vi "PMTRunPulseSet.vi"(3 "error in":errorcluster, 4 "Cluster":T1) -> (0 "error out":errorcluster, 1 "times":u32[][](array[numeric]), 2 "counts":cluster{u32[], u32[], u32[], u32[]})   [LabVIEW 2017]
uses:
  <vilib>/rvi/interface/nirviMethod/nirviMethod.xnode
  <vilib>/rvi/interface/nirviReadWriteControl/nirviReadWriteControl.xnode
  NiFpgaLv.dll
  <vilib>/Utility/error.llb/Error Cluster From Error Code.vi
  <vilib>/rvi/interface/Simulation/niFpgaSimulationCallBeginRW.vi
  <vilib>/rvi/errors/niLvFpgaAdjustHostInterfaceError.vi
  <vilib>/FPGAPlugInAG/Dynamic/niLvFpga_ReadFifo_Dynamic.vi
  <vilib>/rvi/errors/niLvFpgaMergeErrorWithErrorCode.vi
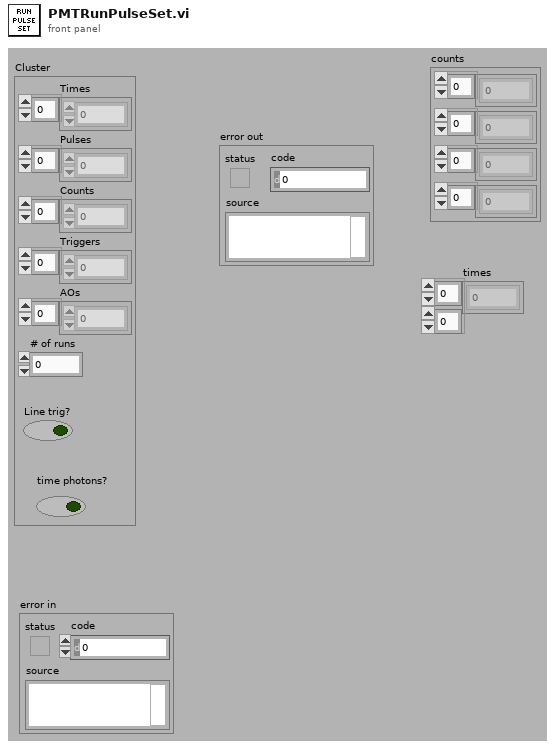
[diagram p1: front panel]
types:
  T1 = cluster{"Times":u32[], "Pulses":u64[], "Counts":u8[], "Triggers":u8[], "AOs":u8[], "# of runs":i32, "Line trig?":bool, "time photons?":bool}
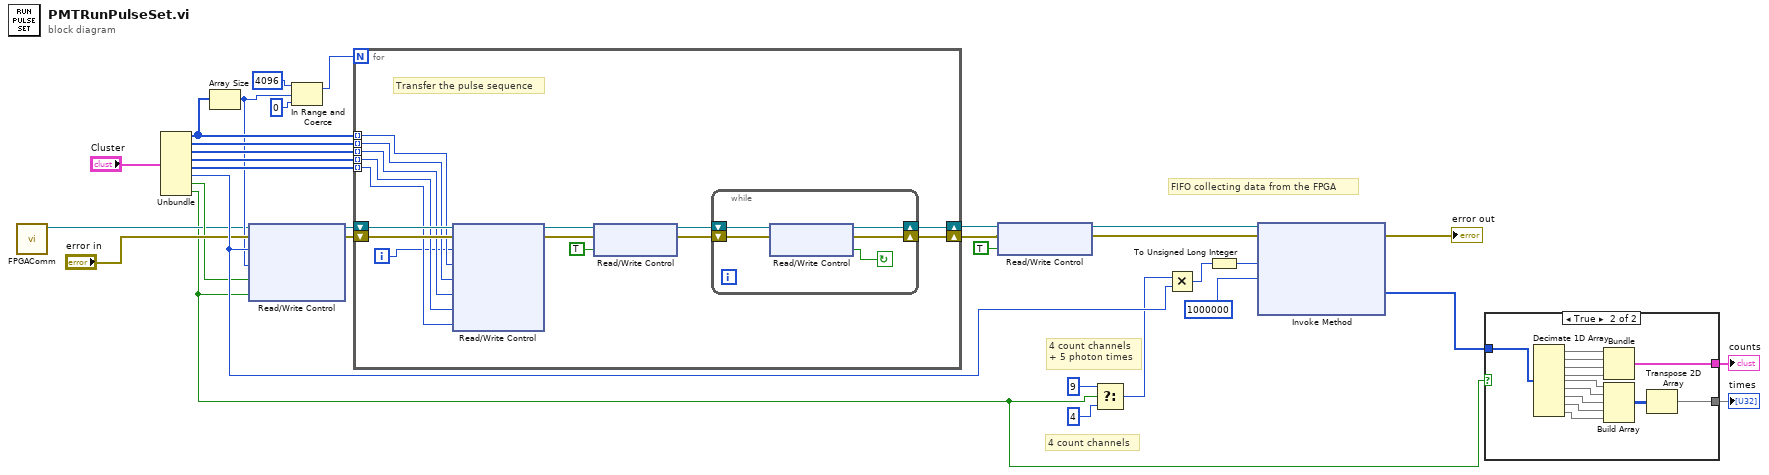
[diagram p0: block diagram]
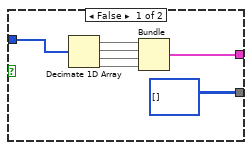
[diagram p2: hidden frame]
diagram:
  # "4 count channels\n+ 5 photon times"
  # "4 count channels"
  # "FIFO collecting data from the FPGA"
  n1 = call "FPGAComm.vi"() -> ("FPGA VI Reference Out 2"=w8:refnum<k20>)  [unwired: 6 in, 1 out]
  n2 = Unbundle("Cluster") -> ("Times"=w11:u32[], "Pulses"=w25:u64[], "Counts"=w26:u8[], "Triggers"=w27:u8[], "AOs"=w28:u8[], "# of runs"=w32:i32, "Line trig?"=w9:bool, "time photons?"=w4:bool)
  n3 = Array Size(array=w11) -> (size(s)=w10:i32)
  n4 = xnode "Read/Write Control"("FPGA VI Reference In"=w8, "error in"="error in", "# of runs"=w32, "# of pulses"=w10, "Line trig?"=w9, "Send photons?"=w4) -> ("FPGA VI Reference Out"=w29:refnum<k20>, "error out"=w31:errorcluster)
  n5 = In Range and Coerce(upper limit=4096, x=w10, lower limit=0) -> (coerced(x)=w24:i32)  [unwired: 1 out]
  n6 = for {
    N: w24 -> [_]
    tunnel: w11 -> [w45] mode=indexing
    tunnel: w25 -> [w44] mode=indexing
    tunnel: w26 -> [w43] mode=indexing
    tunnel: w27 -> [w42] mode=indexing
    tunnel: w28 -> [w41] mode=indexing
    shift-right: [w35] -> w18
    shift-left: w29 -> [w47]
    shift-right: [w34] -> w19
    shift-left: w31 -> [w46]
    i -> [w33]
    # "Transfer the pulse sequence"
    n7 = xnode "Read/Write Control"("FPGA VI Reference In"=w47, "error in"=w46, "pulse number"=w33, "time data"=w45, "digout data"=w44, "count data"=w43, "trigger data"=w42, "AO data"=w41) -> ("FPGA VI Reference Out"=w39:refnum<k20>, "error out"=w38:errorcluster)
    n8 = xnode "Read/Write Control"("FPGA VI Reference In"=w39, "error in"=w38, "data waiting"=TRUE) -> ("FPGA VI Reference Out"=w37:refnum<k20>, "error out"=w36:errorcluster)
    n9 = while {
      shift-right: [w50] -> w35
      shift-left: w37 -> [w52]
      shift-right: [w49] -> w34
      shift-left: w36 -> [w51]
      stop <- w48 continue-if-true
      n10 = xnode "Read/Write Control"("FPGA VI Reference In"=w52, "error in"=w51) -> ("FPGA VI Reference Out"=w50:refnum<k20>, "error out"=w49:errorcluster, "data waiting"=w48:bool)
    }
  }
  n11 = xnode "Read/Write Control"("FPGA VI Reference In"=w18, "error in"=w19, "start sequence"=TRUE) -> ("FPGA VI Reference Out"=w12:refnum<k20>, "error out"=w13:errorcluster)
  n12 = Select(t=9, s=w4, f=4 ("x")) -> (s? t:f=w6:i32)
  n13 = Multiply(x=w6, y=w32) -> (x*y=w15:i32)
  n14 = To Unsigned Long Integer(number=w15) -> (unsigned 32bit integer=w17:u32)
  n15 = xnode "Invoke Method"("FPGA VI Reference In"=w12, "error in"=w13, "Number of Elements"=w17, "Timeout (ms)"=1000000) -> ("error out"=→"error out":errorcluster, "Data"=w3:u32[])  [unwired: 2 out]
  n16 = case shown="True" w4 {
    tunnel: w3 -> [w59 w68]
    tunnel: [w54 w67] -> w2
    tunnel: [u32[][] [] ("transposed array") w60] -> w1
    frame False {
      n17 = Decimate 1D Array(w59) -> (w58:u32[], w57:u32[], w56:u32[], w55:u32[])
      n18 = Bundle(w58, w57, w56, w55) -> (w54:cluster{u32[], u32[], u32[], u32[]})  [unwired: 1 in]
    }
    frame True {
      n19 = Decimate 1D Array(w68) -> (w72:u32[], w71:u32[], w70:u32[], w69:u32[], w66:u32[], w65:u32[], w64:u32[], w63:u32[], w62:u32[])
      n20 = Bundle(w72, w71, w70, w69) -> (w67:cluster{u32[], u32[], u32[], u32[]})  [unwired: 1 in]
      n21 = Build Array(w66, w65, w64, w63, w62) -> (w61:u32[][])
      n22 = Transpose 2D Array(2D array=w61) -> (transposed array=w60:u32[][])
    }
  }
  "counts" <- w2
  "times" <- w1
